vi "Pulse once per interval.vi"(1 "Time (ms)":u32) -> (0 "Boolean":bool)   [LabVIEW 2018]
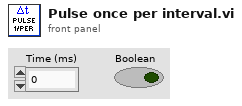
[diagram p1: front panel]
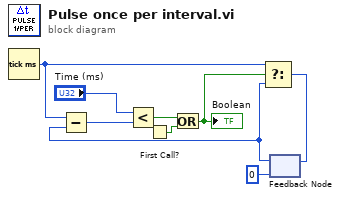
[diagram p0: block diagram]
diagram:
  n1 = Tick Count (ms)() -> (millisecond timer value=w9:u32)
  n2 = First Call?() -> (First Call?: T/F=w3:bool)
  n3 = feedback #1(u32 0 ("y")) -> (w6:u32)
  n4 = Subtract(x=w9, y=w6) -> (x-y=w7:u32)
  n5 = Less?(x="Time (ms)", y=w7) -> (x < y?=w2:bool)
  n6 = Or(x=w2, y=w3) -> (x .or. y?=w1:bool)
  "Boolean" <- w1
  n7 = Select(t=w9, s=w1, f=w6) -> (s? t:f=w5:u32)
  n8 = feedback-in #1(w5) -> ()
